vi "SADD.vi"(0 "refnum in":refnum<vi>, 1 "Key":string, 5 "Members":string[](array[string]), 11 "error in":errorcluster) -> (4 "refnum out":refnum<vi>, 6 "Data":T1, 15 "error out":errorcluster)   [LabVIEW 2020]
uses:
  SubVIs/Controls/redis-data.ctl
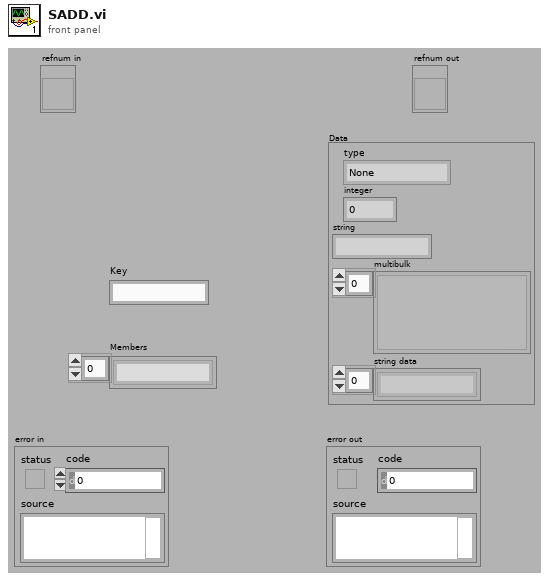
[diagram p1: front panel]
types:
  T1 = typedef "redis-data.ctl" = cluster{"type":enum16{"None", "Error", "Status", "Nil", "Integer", "String", "Multibulk"}, "integer":i64, "string":string, "multibulk":variant[], "string data":string[]}
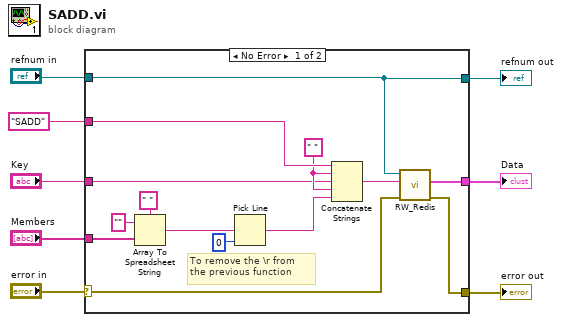
[diagram p0: block diagram]
diagram:
  n1 = case shown="No Error" "error in" {
    selector: "error in" -> [w20 w24]
    tunnel: "Members" -> [w13 _]
    tunnel: "SADD" -> [w22 _]
    tunnel: "refnum in" -> [w9 w23]
    tunnel: [w19 w24] -> w6
    tunnel: [w18 _] -> w3
    tunnel: "Key" -> [w10 _]
    tunnel: [w9 w23] -> w1
    frame No Error {
      w12 = " "
      # "To remove the \\r from\nthe previous function"
      n2 = Array To Spreadsheet String(delimiter (Tab)=" ", array=w13, 3:"" ("format string")) -> (spreadsheet string=w16:string)
      n3 = Pick Line(multi-line string=w16, line index=0) -> (output string=w11:string)  [unwired: 1 in]
      n4 = Concatenate Strings(w22, w12, w10, w12, w11) -> (w21:string)
      n5 = call "RW_Redis.vi"("error in"=w20, "command"=w21, "refnum"=w9) -> ("error out"=w19:errorcluster, "Data"=w18:T1)  [unwired: 7 in]
    }
    frame Error {
    }
  }
  "error out" <- w6
  "refnum out" <- w1
  "Data" <- w3
